vi "ev Frame name.vi"(8 "error in (no error)":errorcluster, 11 "LF2R IDE in":refnum<class "LF2R IDE.lvclass">) -> (0 "error out":errorcluster, 3 "LF2R IDE out":refnum<class "LF2R IDE.lvclass">)   [LabVIEW 2018, in "LF2R IDE.lvlib" / "LF2R IDE.lvclass"]
uses:
  LF2R IDE.lvclass
  LF2R IDE.lvclass/LF2R IDE.ctl
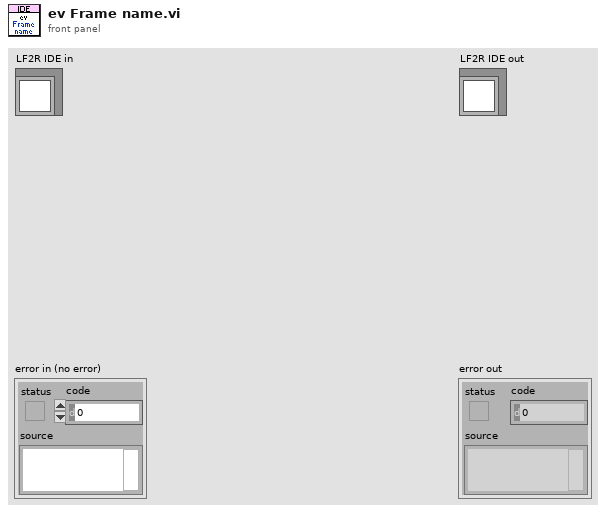
[diagram p1: front panel]
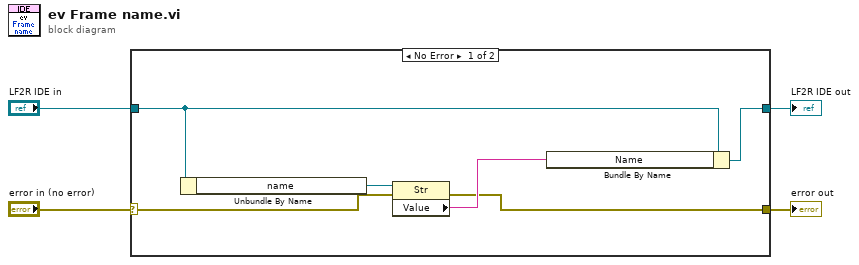
[diagram p0: block diagram]
diagram:
  n1 = case shown="No Error" "error in (no error)" {
    selector: "error in (no error)" -> [w8 w12]
    tunnel: [w5 w12] -> w3
    tunnel: [w7 w11] -> w1
    tunnel: "LF2R IDE in" -> [w10 w11]
    frame No Error {
      n2 = Unbundle By Name(w10) -> ("name"=w9:refnum<vi>)
      n3 = property class="Str"(reference=w9, error in=w8) -> (error out=w5:errorcluster, "Value"=w6:string)  [unwired: 1 out]
      n4 = Bundle By Name(cluster=w10, "Name"=w6) -> (w7:refnum<class "LF2R IDE.lvclass">)
    }
    frame Error {
    }
  }
  "error out" <- w3
  "LF2R IDE out" <- w1
